vi "ByteArray to Variant.vi"(4 "index":i32[](array[numeric]), 6 "Size(s)":i32[](array[numeric]), 8 "error in (no error)":errorcluster, 9 "Data Type":T1, 10 "Endianess":T2, 11 "byte array":u8[](array[numeric])) -> (0 "error out":errorcluster, 3 "Variant":variant)   [LabVIEW 2021, in "Ring Buffer Strict Accessor.lvlib"]
uses:
  Ring Buffer Strict Accessor.lvlib
  Endianess.ctl
  DataType.ctl
  8a60398d-b755-4916-b991-d3a0bc5f0417.vi
  751c3a01-ff04-4836-b7a6-7b574d4a9b81.vi
  221f450a-1b6f-46a4-a2fc-afe85f1524e2.vi
  41001614-cdbd-4ebb-921a-864de9ec47e2.vi
  5546051e-c623-4301-8272-f4bdabd7954b.vi
  5ca96b41-1aac-43f3-81c4-abd3cf1c6587.vi
  7d34a3b6-a7c4-49dd-9cdf-fb0f78c178d5.vi
  d8189c62-4619-451b-9af1-1c592367667c.vi
  ae543023-a94a-4a2d-bef6-e89c8b6f7eb3.vi
  788b2cc3-569e-4ae0-be57-2fef15c96938.vi
  2b477ad7-803c-4946-b2f4-1fc748402100.vi
  098c5dbb-e4d0-4c7a-81ed-dc9b4f9ca07a.vi
  0e7c8b9e-e897-4ed3-8864-39927aea5c8f.vi
  f4fc8823-9e07-4dc6-8a2a-c00e5aad4daa.vi
  4e00dd29-4a4f-4c51-b5d6-93aa465532c5.vi
  5f2f642a-ad03-4c41-b5d5-f276612f3591.vi
  571e8695-7815-4b46-9fe8-94e034d2cc8e.vi
  3d662265-0079-46bb-92db-c9b066d77669.vi
  817a4f5e-2c65-4066-9894-ecba4a0e477b.vi
  3fadb452-1f1f-455e-89f0-d18ad6ef6ba2.vi
  5d6b12d9-691a-45b4-9c34-a3da6780b00a.vi
  9891769e-6c37-4b59-a094-aa89e879cb8b.vi
  <vilib>/Utility/error.llb/Error Cluster From Error Code.vi
  <vilib>/ErrorRing/Error Ring.xnode
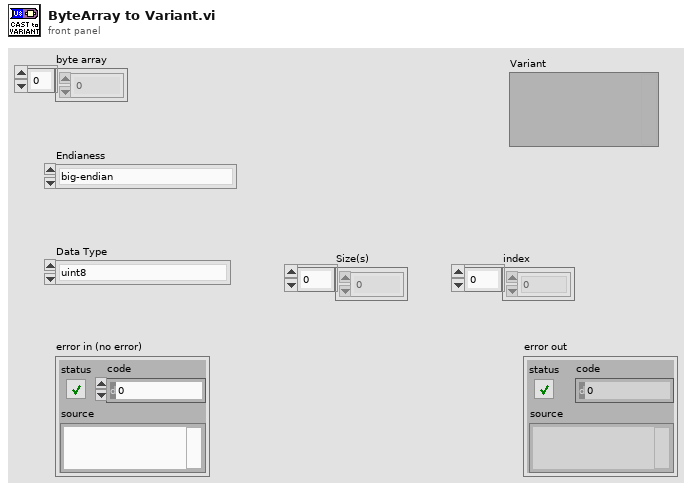
[diagram p1: front panel]
types:
  T1 = typedef "Ring Buffer Strict Accessor.lvlib/DataType.ctl" = enum16{"uint8", "uint16", "uint32", "uint64", "int8", "int16", "int32", "int64", "float", "double", "extended"}
  T2 = typedef "Ring Buffer Strict Accessor.lvlib/Endianess.ctl" = enum16{"big-endian", "little-endian"}
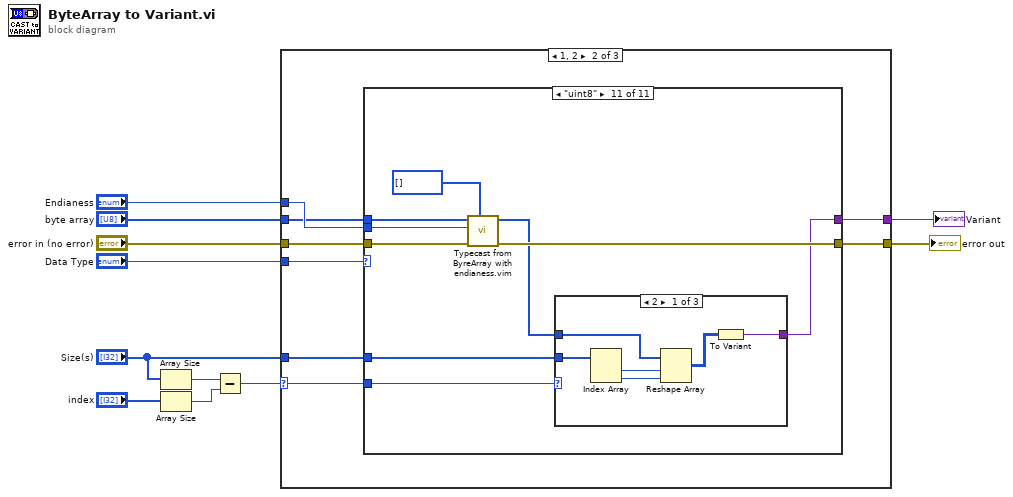
[diagram p0: block diagram]
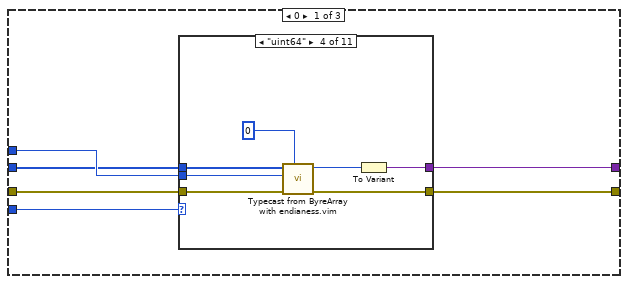
[diagram p2: hidden frame]
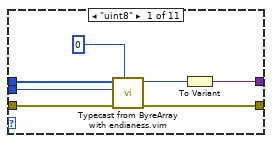
[diagram p3: hidden frame]
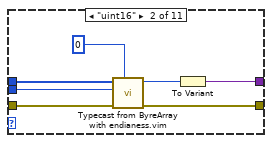
[diagram p4: hidden frame]
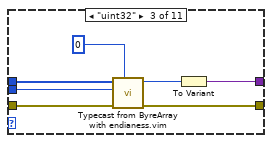
[diagram p5: hidden frame]
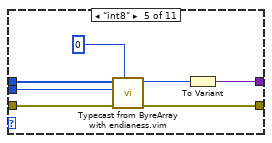
[diagram p6: hidden frame]
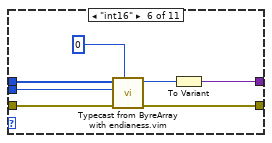
[diagram p7: hidden frame]
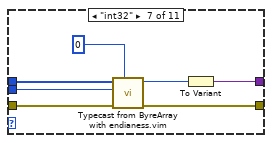
[diagram p8: hidden frame]
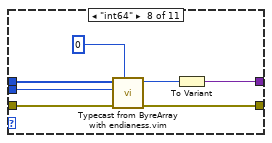
[diagram p9: hidden frame]
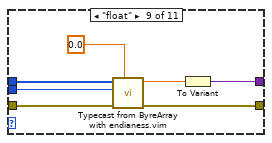
[diagram p10: hidden frame]
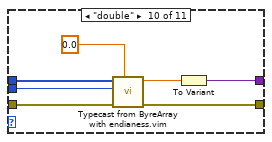
[diagram p11: hidden frame]
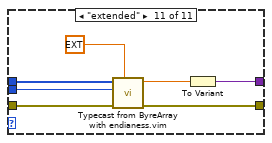
[diagram p12: hidden frame]
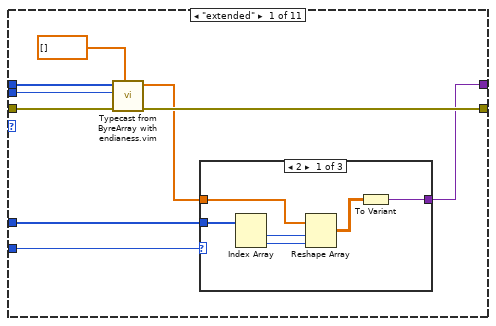
[diagram p13: hidden frame]
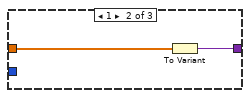
[diagram p14: hidden frame]
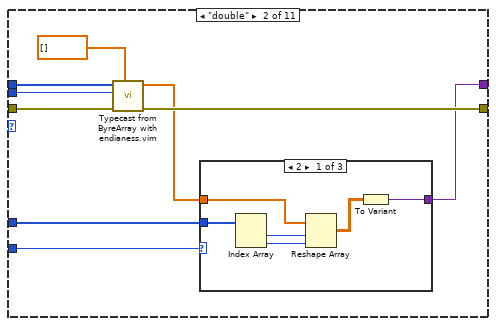
[diagram p16: hidden frame]
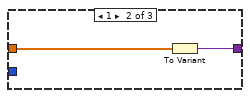
[diagram p17: hidden frame]
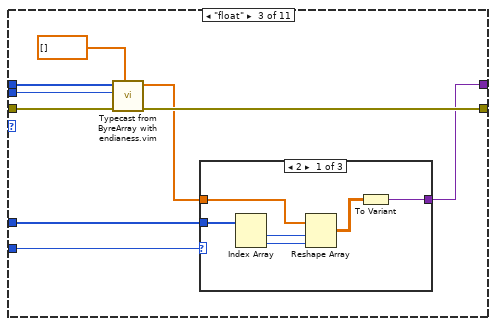
[diagram p19: hidden frame]
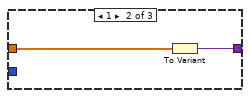
[diagram p20: hidden frame]
diagram:
  n1 = Array Size(array="Size(s)") -> (size(s)=w3:i32)
  n2 = Array Size(array="index") -> (size(s)=w2:i32)
  n3 = Subtract(x=w3, y=w2) -> (x-y=w1:i32)
  n4 = case shown="1, 2" w1 {
    selector: w1 -> [_ w96 w293]
    tunnel: "Endianess" -> [w17 w101 _]
    tunnel: "byte array" -> [w16 w100 _]
    tunnel: "error in (no error)" -> [w15 w99 w292]
    tunnel: "Data Type" -> [w14 w98 _]
    tunnel: [w13 w95 _] -> w7
    tunnel: [w12 w102 w290] -> w6
    tunnel: "Size(s)" -> [_ w97 _]
    frame 0 {
      n5 = case shown="\"uint64\"" w14 {
        tunnel: w16 -> [w23 w30 w37 w44 w51 w58 w65 w72 w79 w87 w93]
        tunnel: w17 -> [w22 w29 w36 w43 w50 w57 w64 w71 w78 w86 w92]
        tunnel: w15 -> [w21 w28 w35 w42 w49 w56 w63 w70 w77 w84 w91]
        tunnel: [w20 w27 w34 w41 w48 w55 w62 w69 w76 w83 w90] -> w12
        tunnel: [w18 w25 w32 w39 w46 w53 w60 w67 w74 w81 w88] -> w13
        frame "uint8" {
          n6 = call "Typecast from ByreArray with endianess.vim"("data type"=u8 0, "error in (no error)"=w21, "Endianess"=w22, "byte array"=w23) -> ("error out"=w20:errorcluster, "data"=w19:u8)  [unwired: 6 in]
          n7 = To Variant(anything=w19) -> (Variant=w18:variant)
        }
        frame "uint16" {
          n8 = call "Typecast from ByreArray with endianess.vim"("data type"=u16 0, "error in (no error)"=w28, "Endianess"=w29, "byte array"=w30) -> ("error out"=w27:errorcluster, "data"=w26:u16)  [unwired: 6 in]
          n9 = To Variant(anything=w26) -> (Variant=w25:variant)
        }
        frame "uint32" {
          n10 = call "Typecast from ByreArray with endianess.vim"("data type"=u32 0, "error in (no error)"=w35, "Endianess"=w36, "byte array"=w37) -> ("error out"=w34:errorcluster, "data"=w33:u32)  [unwired: 6 in]
          n11 = To Variant(anything=w33) -> (Variant=w32:variant)
        }
        frame "uint64" {
          n12 = call "Typecast from ByreArray with endianess.vim"("data type"=u64 0, "error in (no error)"=w42, "Endianess"=w43, "byte array"=w44) -> ("error out"=w41:errorcluster, "data"=w40:u64)  [unwired: 6 in]
          n13 = To Variant(anything=w40) -> (Variant=w39:variant)
        }
        frame "int8" {
          n14 = call "Typecast from ByreArray with endianess.vim"("data type"=i8 0, "error in (no error)"=w49, "Endianess"=w50, "byte array"=w51) -> ("error out"=w48:errorcluster, "data"=w47:i8)  [unwired: 6 in]
          n15 = To Variant(anything=w47) -> (Variant=w46:variant)
        }
        frame "int16" {
          n16 = call "Typecast from ByreArray with endianess.vim"("data type"=i16 0, "error in (no error)"=w56, "Endianess"=w57, "byte array"=w58) -> ("error out"=w55:errorcluster, "data"=w54:i16)  [unwired: 6 in]
          n17 = To Variant(anything=w54) -> (Variant=w53:variant)
        }
        frame "int32" {
          n18 = call "Typecast from ByreArray with endianess.vim"("data type"=0, "error in (no error)"=w63, "Endianess"=w64, "byte array"=w65) -> ("error out"=w62:errorcluster, "data"=w61:i32)  [unwired: 6 in]
          n19 = To Variant(anything=w61) -> (Variant=w60:variant)
        }
        frame "int64" {
          n20 = call "Typecast from ByreArray with endianess.vim"("data type"=i64 0, "error in (no error)"=w70, "Endianess"=w71, "byte array"=w72) -> ("error out"=w69:errorcluster, "data"=w68:i64)  [unwired: 6 in]
          n21 = To Variant(anything=w68) -> (Variant=w67:variant)
        }
        frame "float" {
          n22 = call "Typecast from ByreArray with endianess.vim"("data type"=sgl 0.0, "error in (no error)"=w77, "Endianess"=w78, "byte array"=w79) -> ("error out"=w76:errorcluster, "data"=w75:sgl)  [unwired: 6 in]
          n23 = To Variant(anything=w75) -> (Variant=w74:variant)
        }
        frame "double" {
          n24 = call "Typecast from ByreArray with endianess.vim"("data type"=0.0 ("Numeric"), "error in (no error)"=w84, "Endianess"=w86, "byte array"=w87) -> ("error out"=w83:errorcluster, "data"=w82:dbl)  [unwired: 6 in]
          n25 = To Variant(anything=w82) -> (Variant=w81:variant)
        }
        frame "extended" {
          n26 = call "Typecast from ByreArray with endianess.vim"("data type"=ext 0.0, "error in (no error)"=w91, "Endianess"=w92, "byte array"=w93) -> ("error out"=w90:errorcluster, "data"=w89:ext)  [unwired: 6 in]
          n27 = To Variant(anything=w89) -> (Variant=w88:variant)
        }
      }
    }
    frame 1, 2 {
      n28 = case shown="\"uint8\"" w98 {
        tunnel: w100 -> [w110 w127 w144 w161 w178 w195 w212 w229 w246 w263 w280]
        tunnel: w101 -> [w109 w126 w143 w160 w177 w194 w211 w228 w245 w262 w279]
        tunnel: [w104 w121 w138 w155 w172 w189 w206 w223 w240 w257 w274] -> w95
        tunnel: w99 -> [w108 w125 w142 w159 w176 w193 w210 w227 w244 w261 w278]
        tunnel: [w107 w124 w141 w158 w175 w192 w209 w226 w243 w260 w277] -> w102
        tunnel: w97 -> [w105 w122 w139 w156 w173 w190 w207 w224 w241 w258 w275]
        tunnel: w96 -> [w103 w120 w137 w154 w171 w188 w205 w222 w239 w256 w273]
        frame "extended" {
          n29 = call "Typecast from ByreArray with endianess.vim"("data type"=ext[] [], "error in (no error)"=w108, "Endianess"=w109, "byte array"=w110) -> ("error out"=w107:errorcluster, "data"=w106:ext[])  [unwired: 6 in]
          n30 = case shown="2" w103 {
            tunnel: w106 -> [w117 w118 _]
            tunnel: w105 -> [w116 _ _]
            tunnel: [w112 w119 _] -> w104
            frame 2 {
              n31 = Index Array(array=w116) -> (element #1=w115:i32, element #2=w114:i32)  [unwired: 2 in]
              n32 = Reshape Array(w117, w115, w114) -> (w113:ext[][])
              n33 = To Variant(anything=w113) -> (Variant=w112:variant)
            }
            frame 1 {
              n34 = To Variant(anything=w118) -> (Variant=w119:variant)
            }
            frame Default {
            }
          }
        }
        frame "double" {
          n35 = call "Typecast from ByreArray with endianess.vim"("data type"=dbl[] [], "error in (no error)"=w125, "Endianess"=w126, "byte array"=w127) -> ("error out"=w124:errorcluster, "data"=w123:dbl[])  [unwired: 6 in]
          n36 = case shown="2" w120 {
            tunnel: w123 -> [w134 w135 _]
            tunnel: w122 -> [w133 _ _]
            tunnel: [w129 w136 _] -> w121
            frame 2 {
              n37 = Index Array(array=w133) -> (element #1=w132:i32, element #2=w131:i32)  [unwired: 2 in]
              n38 = Reshape Array(w134, w132, w131) -> (w130:dbl[][])
              n39 = To Variant(anything=w130) -> (Variant=w129:variant)
            }
            frame 1 {
              n40 = To Variant(anything=w135) -> (Variant=w136:variant)
            }
            frame Default {
            }
          }
        }
        frame "float" {
          n41 = call "Typecast from ByreArray with endianess.vim"("data type"=sgl[] [], "error in (no error)"=w142, "Endianess"=w143, "byte array"=w144) -> ("error out"=w141:errorcluster, "data"=w140:sgl[])  [unwired: 6 in]
          n42 = case shown="2" w137 {
            tunnel: w140 -> [w151 w152 _]
            tunnel: w139 -> [w150 _ _]
            tunnel: [w146 w153 _] -> w138
            frame 2 {
              n43 = Index Array(array=w150) -> (element #1=w149:i32, element #2=w148:i32)  [unwired: 2 in]
              n44 = Reshape Array(w151, w149, w148) -> (w147:sgl[][])
              n45 = To Variant(anything=w147) -> (Variant=w146:variant)
            }
            frame 1 {
              n46 = To Variant(anything=w152) -> (Variant=w153:variant)
            }
            frame Default {
            }
          }
        }
        frame "int64" {
          n47 = call "Typecast from ByreArray with endianess.vim"("data type"=i64[] [], "error in (no error)"=w159, "Endianess"=w160, "byte array"=w161) -> ("error out"=w158:errorcluster, "data"=w157:i64[])  [unwired: 6 in]
          n48 = case shown="2" w154 {
            tunnel: w157 -> [w168 w169 _]
            tunnel: w156 -> [w167 _ _]
            tunnel: [w163 w170 _] -> w155
            frame 2 {
              n49 = Index Array(array=w167) -> (element #1=w166:i32, element #2=w165:i32)  [unwired: 2 in]
              n50 = Reshape Array(w168, w166, w165) -> (w164:i64[][])
              n51 = To Variant(anything=w164) -> (Variant=w163:variant)
            }
            frame 1 {
              n52 = To Variant(anything=w169) -> (Variant=w170:variant)
            }
            frame Default {
            }
          }
        }
        frame "int32" {
          n53 = call "Typecast from ByreArray with endianess.vim"("data type"=i32[] [], "error in (no error)"=w176, "Endianess"=w177, "byte array"=w178) -> ("error out"=w175:errorcluster, "data"=w174:i32[])  [unwired: 6 in]
          n54 = case shown="2" w171 {
            tunnel: w174 -> [w185 w186 _]
            tunnel: w173 -> [w184 _ _]
            tunnel: [w180 w187 _] -> w172
            frame 2 {
              n55 = Index Array(array=w184) -> (element #1=w183:i32, element #2=w182:i32)  [unwired: 2 in]
              n56 = Reshape Array(w185, w183, w182) -> (w181:i32[][])
              n57 = To Variant(anything=w181) -> (Variant=w180:variant)
            }
            frame 1 {
              n58 = To Variant(anything=w186) -> (Variant=w187:variant)
            }
            frame Default {
            }
          }
        }
        frame "int16" {
          n59 = call "Typecast from ByreArray with endianess.vim"("data type"=i16[] [], "error in (no error)"=w193, "Endianess"=w194, "byte array"=w195) -> ("error out"=w192:errorcluster, "data"=w191:i16[])  [unwired: 6 in]
          n60 = case shown="2" w188 {
            tunnel: w191 -> [w202 w203 _]
            tunnel: w190 -> [w201 _ _]
            tunnel: [w197 w204 _] -> w189
            frame 2 {
              n61 = Index Array(array=w201) -> (element #1=w200:i32, element #2=w199:i32)  [unwired: 2 in]
              n62 = Reshape Array(w202, w200, w199) -> (w198:i16[][])
              n63 = To Variant(anything=w198) -> (Variant=w197:variant)
            }
            frame 1 {
              n64 = To Variant(anything=w203) -> (Variant=w204:variant)
            }
            frame Default {
            }
          }
        }
        frame "int8" {
          n65 = call "Typecast from ByreArray with endianess.vim"("data type"=i8[] [], "error in (no error)"=w210, "Endianess"=w211, "byte array"=w212) -> ("error out"=w209:errorcluster, "data"=w208:i8[])  [unwired: 6 in]
          n66 = case shown="2" w205 {
            tunnel: w208 -> [w219 w220 _]
            tunnel: w207 -> [w218 _ _]
            tunnel: [w214 w221 _] -> w206
            frame 2 {
              n67 = Index Array(array=w218) -> (element #1=w217:i32, element #2=w216:i32)  [unwired: 2 in]
              n68 = Reshape Array(w219, w217, w216) -> (w215:i8[][])
              n69 = To Variant(anything=w215) -> (Variant=w214:variant)
            }
            frame 1 {
              n70 = To Variant(anything=w220) -> (Variant=w221:variant)
            }
            frame Default {
            }
          }
        }
        frame "uint64" {
          n71 = call "Typecast from ByreArray with endianess.vim"("data type"=u64[] [], "error in (no error)"=w227, "Endianess"=w228, "byte array"=w229) -> ("error out"=w226:errorcluster, "data"=w225:u64[])  [unwired: 6 in]
          n72 = case shown="2" w222 {
            tunnel: w225 -> [w236 w237 _]
            tunnel: w224 -> [w235 _ _]
            tunnel: [w231 w238 _] -> w223
            frame 2 {
              n73 = Index Array(array=w235) -> (element #1=w234:i32, element #2=w233:i32)  [unwired: 2 in]
              n74 = Reshape Array(w236, w234, w233) -> (w232:u64[][])
              n75 = To Variant(anything=w232) -> (Variant=w231:variant)
            }
            frame 1 {
              n76 = To Variant(anything=w237) -> (Variant=w238:variant)
            }
            frame Default {
            }
          }
        }
        frame "uint32" {
          n77 = call "Typecast from ByreArray with endianess.vim"("data type"=u32[] [], "error in (no error)"=w244, "Endianess"=w245, "byte array"=w246) -> ("error out"=w243:errorcluster, "data"=w242:u32[])  [unwired: 6 in]
          n78 = case shown="2" w239 {
            tunnel: w242 -> [w253 w254 _]
            tunnel: w241 -> [w252 _ _]
            tunnel: [w248 w255 _] -> w240
            frame 2 {
              n79 = Index Array(array=w252) -> (element #1=w251:i32, element #2=w250:i32)  [unwired: 2 in]
              n80 = Reshape Array(w253, w251, w250) -> (w249:u32[][])
              n81 = To Variant(anything=w249) -> (Variant=w248:variant)
            }
            frame 1 {
              n82 = To Variant(anything=w254) -> (Variant=w255:variant)
            }
            frame Default {
            }
          }
        }
        frame "uint16" {
          n83 = call "Typecast from ByreArray with endianess.vim"("data type"=u16[] [], "error in (no error)"=w261, "Endianess"=w262, "byte array"=w263) -> ("error out"=w260:errorcluster, "data"=w259:u16[])  [unwired: 6 in]
          n84 = case shown="2" w256 {
            tunnel: w259 -> [w270 w271 _]
            tunnel: w258 -> [w269 _ _]
            tunnel: [w265 w272 _] -> w257
            frame 2 {
              n85 = Index Array(array=w269) -> (element #1=w268:i32, element #2=w267:i32)  [unwired: 2 in]
              n86 = Reshape Array(w270, w268, w267) -> (w266:u16[][])
              n87 = To Variant(anything=w266) -> (Variant=w265:variant)
            }
            frame 1 {
              n88 = To Variant(anything=w271) -> (Variant=w272:variant)
            }
            frame Default {
            }
          }
        }
        frame "uint8" {
          n89 = call "Typecast from ByreArray with endianess.vim"("data type"=u8[] [], "error in (no error)"=w278, "Endianess"=w279, "byte array"=w280) -> ("error out"=w277:errorcluster, "data"=w276:u8[])  [unwired: 6 in]
          n90 = case shown="2" w273 {
            tunnel: w276 -> [w287 w288 _]
            tunnel: w275 -> [w286 _ _]
            tunnel: [w282 w289 _] -> w274
            frame 2 {
              n91 = Index Array(array=w286) -> (element #1=w285:i32, element #2=w284:i32)  [unwired: 2 in]
              n92 = Reshape Array(w287, w285, w284) -> (w283:u8[][])
              n93 = To Variant(anything=w283) -> (Variant=w282:variant)
            }
            frame 1 {
              n94 = To Variant(anything=w288) -> (Variant=w289:variant)
            }
            frame Default {
            }
          }
        }
      }
    }
    frame Default {
      n95 = xnode "Error Ring"("parameter 0"=w293) -> ("error out"=w291:errorcluster)
      n96 = Merge Errors(w292, w291) -> (w290:errorcluster)
    }
  }
  "error out" <- w6
  "Variant" <- w7
